vi "Counts in Last Second.vi"() -> (1 "Counts In Last Second":i32)   [LabVIEW 2021]
uses:
  <vilib>/Utility/High Resolution Relative Seconds.vi
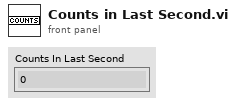
[diagram p1: front panel]
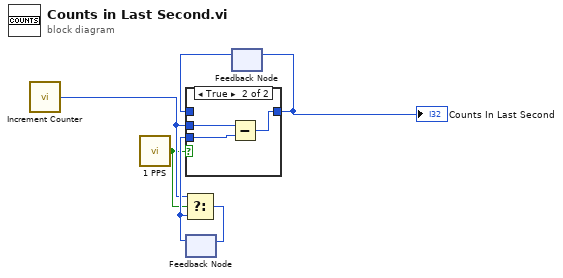
[diagram p0: block diagram]
diagram:
  n1 = call "Increment Counter.vi"() -> ("Count"=w3:i32)  [unwired: 5 in]
  n2 = call "1 PPS.vi"() -> ("1PPS"=w2:bool)  [unwired: 14 in, 1 out]
  n3 = feedback #1() -> (w4:i32)  [unwired: 1 in]
  n4 = Select(t=w3, s=w2, f=w4) -> (s? t:f=w1:i32)
  n5 = feedback-in #1(w1) -> ()
  n6 = feedback #2() -> (w6:i32)  [unwired: 1 in]
  n7 = case shown="True" w2 {
    tunnel: w3 -> [_ w10]
    tunnel: w4 -> [_ w9]
    tunnel: [w7 w8] -> w5
    tunnel: w6 -> [w7 _]
    frame False {
    }
    frame True {
      n8 = Subtract(x=w10, y=w9) -> (x-y=w8:i32)
    }
  }
  "Counts In Last Second" <- w5
  n9 = feedback-in #2(w5) -> ()
